vi "Stop.vi"() -> ()   [LabVIEW 2016]
panel:
  in  "Stop":bool
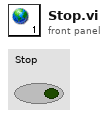
[diagram p1: front panel]
diagram:
